vi "Report Get Distinct Grids.vi"(11 "All Grids":i32[](array[numeric])) -> (3 "Distinct Grid":i32[](array[numeric]))   [LabVIEW 2020]
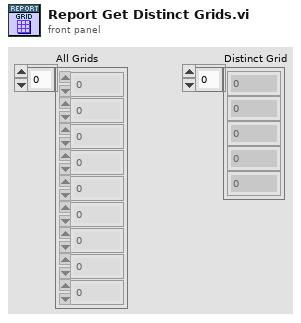
[diagram p1: front panel]
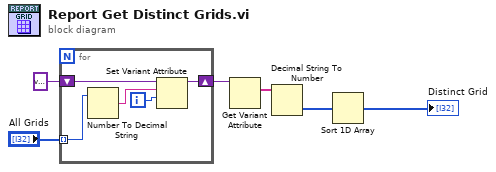
[diagram p0: block diagram]
diagram:
  n1 = for {
    tunnel: "All Grids" -> [w11] mode=indexing
    shift-right: [w8] -> w4
    shift-left: variant -> [w7]
    i -> [w9]
    n2 = Number To Decimal String(number=w11) -> (decimal integer string=w10:string)  [unwired: 1 in]
    n3 = Set Variant Attribute(Variant=w7, name=w10, value=w9) -> (Variant out=w8:variant)  [unwired: 1 in, 2 out]
  }
  n4 = Get Variant Attribute(Variant=w4) -> (names=w5:string[])  [unwired: 3 in, 3 out]
  n5 = Decimal String To Number(string=w5) -> (number=w2:i32[])  [unwired: 2 in, 1 out]
  n6 = Sort 1D Array(array=w2) -> (sorted array=→"Distinct Grid":i32[])
